vi "Threshold Setting.vi"() -> ()   [LabVIEW 2022 SP3]
panel:
  in  "V1 Y2":dbl
  in  "V1 X2":dbl
  in  "V1 H V 2":dbl
  in  "V1 L V 2":dbl
  in  "V1 H A2":dbl
  in  "V1 L A2":dbl
  in  "Save":bool
  in  "V1 Y":dbl
  in  "V1 X":dbl
  in  "V1 H R":dbl
  in  "V1 L R":dbl
  in  "V1 H C":dbl
  in  "V1 L C":dbl
  in  "V1 H A":dbl
  in  "V1 L A":dbl
  in  "V1 H V":dbl
  in  "V1 L V":dbl
  in  "Button":bool
  # "V"
  # "V"
  # "A"
  # "A"
  # "A"
  # "A"
  # "ohm"
  # "ohm"
  # "V"
  # "V"
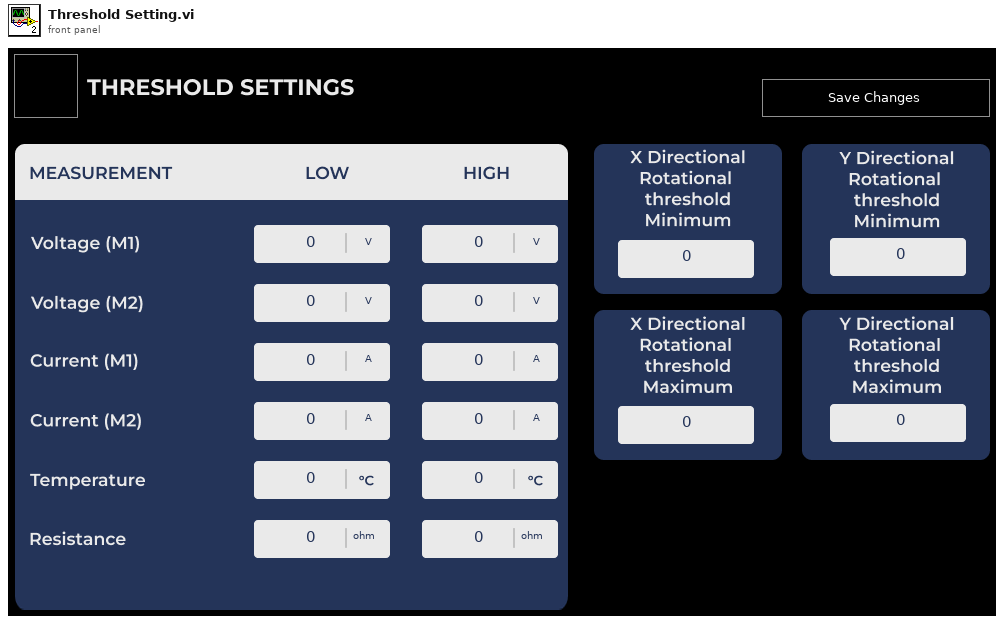
[diagram p1: front panel]
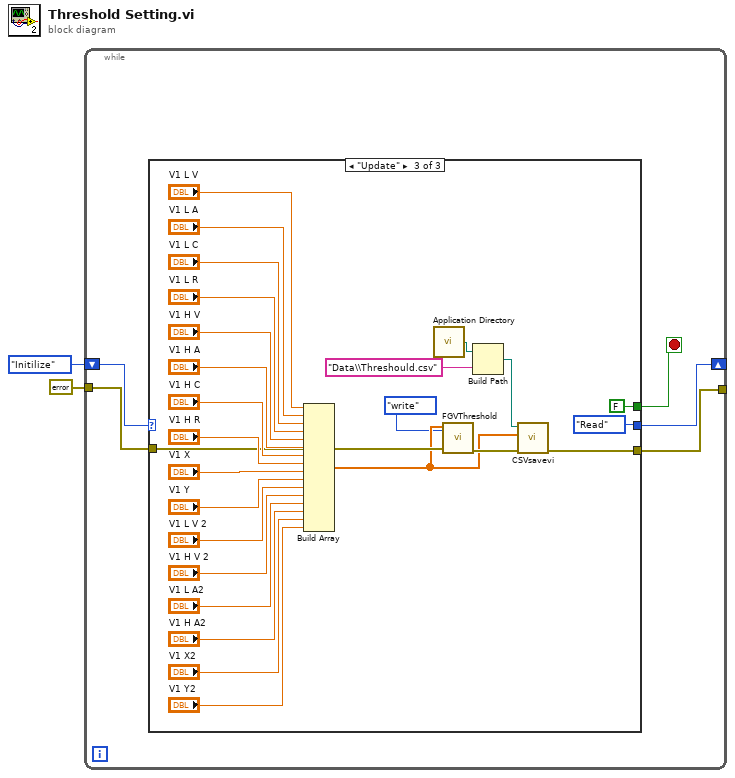
[diagram p0: block diagram]
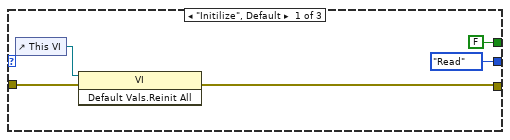
[diagram p2: hidden frame]
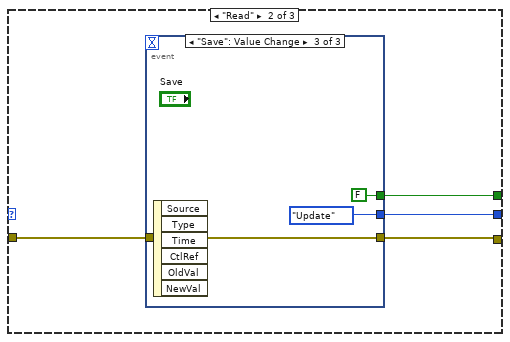
[diagram p3: hidden frame]
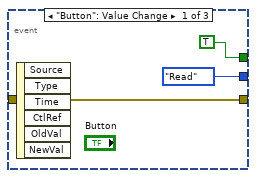
[diagram p4: hidden frame]
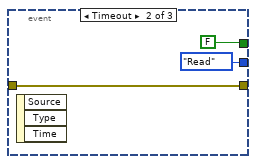
[diagram p5: hidden frame]
diagram:
  n1 = while {
    shift-right: [w6] -> _
    shift-left: enum16{"Initilize", "Read", "Update", "Exit"}."Initilize" -> [w7]
    tunnel: errorcluster {"status"=FALSE, "code"=0, "source"=""} ("error in (no error)") -> [w4]
    tunnel: [w3] -> _
    stop <- w5 stop-if-true
    n2 = case shown="\"Update\"" w7 {
      tunnel: [enum16{"Initilize", "Read", "Update", "Exit"}."Read" w16 enum16{"Initilize", "Read", "Update", "Exit"}."Read"] -> w6
      tunnel: [FALSE w13 FALSE] -> w5
      tunnel: w4 -> [w9 w15 w35]
      tunnel: [w8 w14 w48] -> w3
      frame "Initilize", Default {
        n3 = control-ref of="This VI"() -> (w10:refnum<vi>)
        n4 = invoke class="VI" method="Default Vals.Reinit All"(reference=w10, error in=w9) -> (error out=w8:errorcluster)  [unwired: 1 in, 2 out]
      }
      frame "Read" {
        n5 = event shown="[2] \"Save\": Value Change" {
          selector: _ -> [_ _ _]
          dyn-events: _ -> [_ _ _]
          timeout: _ -> [_ _ _]
          tunnel: [enum16{"Initilize", "Read", "Update", "Exit"}."Read" enum16{"Initilize", "Read", "Update", "Exit"}."Read" enum16{"Initilize", "Read", "Update", "Exit"}."Update"] -> w16
          tunnel: w15 -> [w18 w20 w25]
          tunnel: [w18 w20 w25] -> w14
          tunnel: [TRUE FALSE FALSE] -> w13
          event "Button": Value Change {
            n6 = event-data() -> ()  [unwired: 1 in, 6 out]
          }
          event Timeout {
            n7 = event-data() -> ()  [unwired: 1 in, 3 out]
          }
          event "Save": Value Change {
            n8 = event-data() -> ()  [unwired: 1 in, 6 out]
          }
        }
      }
      frame "Update" {
        n9 = Build Array("V1 L V", "V1 L A", "V1 L C", "V1 L R", "V1 H V", "V1 H A", "V1 H C", "V1 H R", "V1 X", "V1 Y", "V1 L V 2", "V1 H V 2", "V1 L A2", "V1 H A2", "V1 X2", "V1 Y2") -> (w33:dbl[])
        n10 = call <vilib>:"Application Directory.vi"() -> ("Application Directory"=w50:path)
        n11 = call "FGVThreshold.vi"("Enum"=enum16{"write", "read"}."write", "error in (no error)"=w35, "appended array 2"=w33) -> ("error in (no error) 2"=w34:errorcluster)  [unwired: 7 in, 1 out]
        n12 = Build Path(base path=w50, name or relative path="Data\\Threshould.csv") -> (appended path=w51:path)
        n13 = call "CSVsavevi.vi"("error in (no error)"=w34, "Input array"=w33, "file path (dialog if empty)"=w51) -> ("error out"=w48:errorcluster)  [unwired: 8 in]
      }
    }
  }
